vi "Message De-Q.vi"(7 "timeout [ms]":i32=100, 8 "error in":errorcluster, 10 "timeout cmd":string="Message Timeout") -> (0 "error out":errorcluster, 1 "Payload":variant, 2 "Command":string, 3 "Message Q Type":T1)   [LabVIEW 2020, in "Hardware.lvlib"]
doc: "DEqueue a message for this component."
uses:
  Hardware.lvlib
  Message Type.ctl
  Message FGV Actions.ctl
panel:
  out "# elements in queue":i32
  out "timed out?":bool
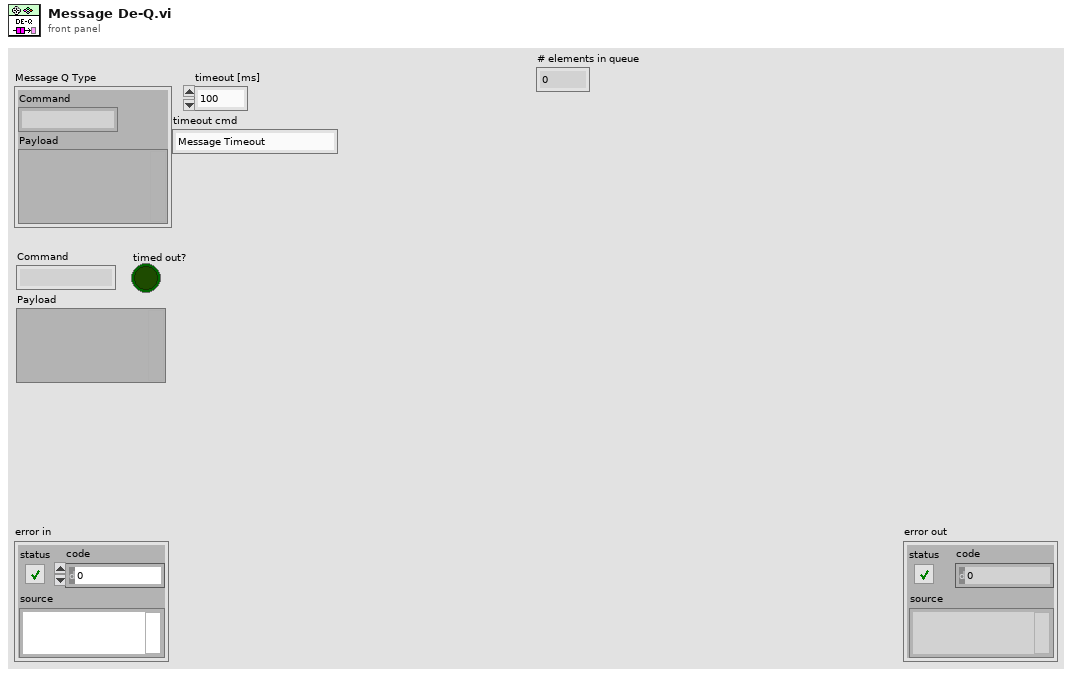
[diagram p1: front panel]
types:
  T1 = typedef "Hardware.lvlib/Message Type.ctl" = cluster{"Command":string, "Payload":variant}
  T2 = typedef "Hardware.lvlib/Message FGV Actions.ctl" = enum16{"Get", "Obtain", "Release", "Flush"}
  T3 = typedef "Component Template.lvlib/Message Q Type.ctl" = cluster{"Command":string, "Payload":variant}
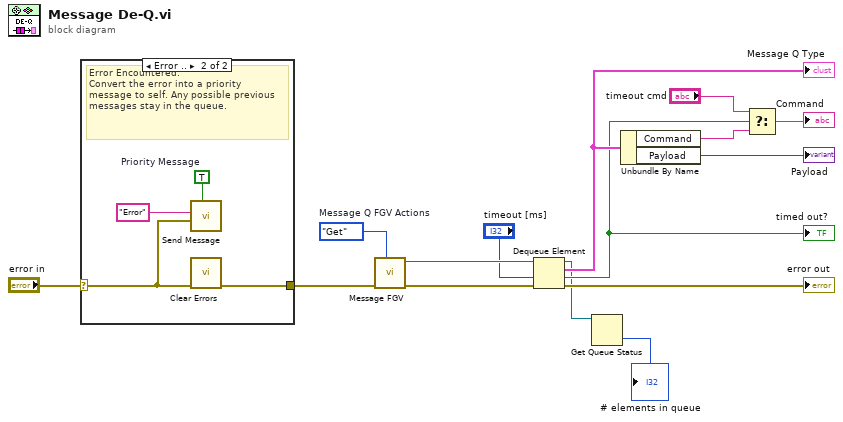
[diagram p0: block diagram]
diagram:
  w14 = Message_FGV_Actions."Get"  # Message Q FGV Actions
  n1 = case shown="Error .." "error in" {
    selector: "error in" -> [w16 w17]
    tunnel: [w16 w18] -> w9
    frame No Error {
    }
    frame Error {
      w19 = TRUE  # Priority Message
      # "Error Encountered.\nConvert the error into a priority message to self. Any possible previous messages stay in the queue."
      n2 = call "Send Message.vi"("Priority Message"=w19, "Payload"=w17, "Command"="Error") -> ()  [unwired: 8 in, 1 out]
      n3 = call <vilib>:"Clear Errors.vi"("error in (no error)"=w17) -> ("error out"=w18:errorcluster)  [unwired: 5 in, 1 out]
    }
  }
  n4 = call "Message FGV.vi"("Message Q FGV Actions"=w14, "error in"=w9) -> ("error out"=w15:errorcluster, "queue ref out"=w12:refnum<queue>)  [unwired: 6 in, 2 out]
  n5 = Dequeue Element(queue=w12, timeout in ms (-1)="timeout [ms]", error in (no error)=w15) -> (queue out=w2:refnum<queue>, element=w11:T3, timed out?=w3:bool, error out=→"error out":errorcluster)
  "Message Q Type" <- w11
  "timed out?" <- w3
  n6 = Get Queue Status(queue=w2) -> (# elements in queue=→"# elements in queue":i32)  [unwired: 2 in, 7 out]
  n7 = Unbundle By Name(w11) -> ("Command"=w5:string, "Payload"=→"Payload":variant)
  n8 = Select(t="timeout cmd", s=w3, f=w5) -> (s? t:f=→"Command":string)
